vi "COMN-RS232_XBEE_RPI.vi"() -> ()   [LabVIEW 2020]
uses:
  <vilib>/Instr/_visa.llb/VISA Configure Serial Port (Instr).vi
panel:
  out "0_HORA":string
  in  "Enable Termination\nChar (T)":bool=TRUE
  in  "termination char\n(0xA = '\\n' = LF)":u8=10 format="%.0x"
  in  "flow control (0:none)":u16(ring) items=["None", "XON/XOFF", "RTS/CTS", "XON/XOFF & RTS/CTS", "DTR/DSR", "XON/XOFF & DTR/DSR"]
  in  "timeout (10sec)":u32=10000
  in  "stop bits (10: 1 bit)":u16(ring)=10 items=["1.0"=10, "1.5"=15, "2.0"=20]
  in  "parity (0:none)":enum16{"None", "Odd", "Even", "Mark", "Space"}(ring)
  in  "data bits (8)":u16=8 min=5 max=8 step=1
  in  "baud rate (9600)":u32=9600
  in  "VISA resource name":refnum<visa-resource-name>
  in  "stop":bool
  out "codigo":bool
  out "mensj_recib":bool
  out "error recib":errorcluster
  out "PUERTO_COM":refnum<visa-resource-name>
  in  "Boton_Recibir":bool
  out "Text_Recibir":string
  # "COMUNICACIÓN RS232 RPI-XBEE-PC"
  # "TEXTO A RECIBIR"
  # "(c)2021"
  # "ANDRES R. PHILIPPS BENITEZ"
  # "HABILITAR \nCARACTER DE\nTERMINACIÓN"
  # "CARACTER DE\nTERMINACION"
  # "TIMEOUT"
  # "CONTROL DE FLUJO"
  # "BITS DATOS"
  # "PARIDAD"
  # "BITS DE STOP"
  # "BAUDIOS"
  # "PUERTO COM"
  # "CÓDIGO"
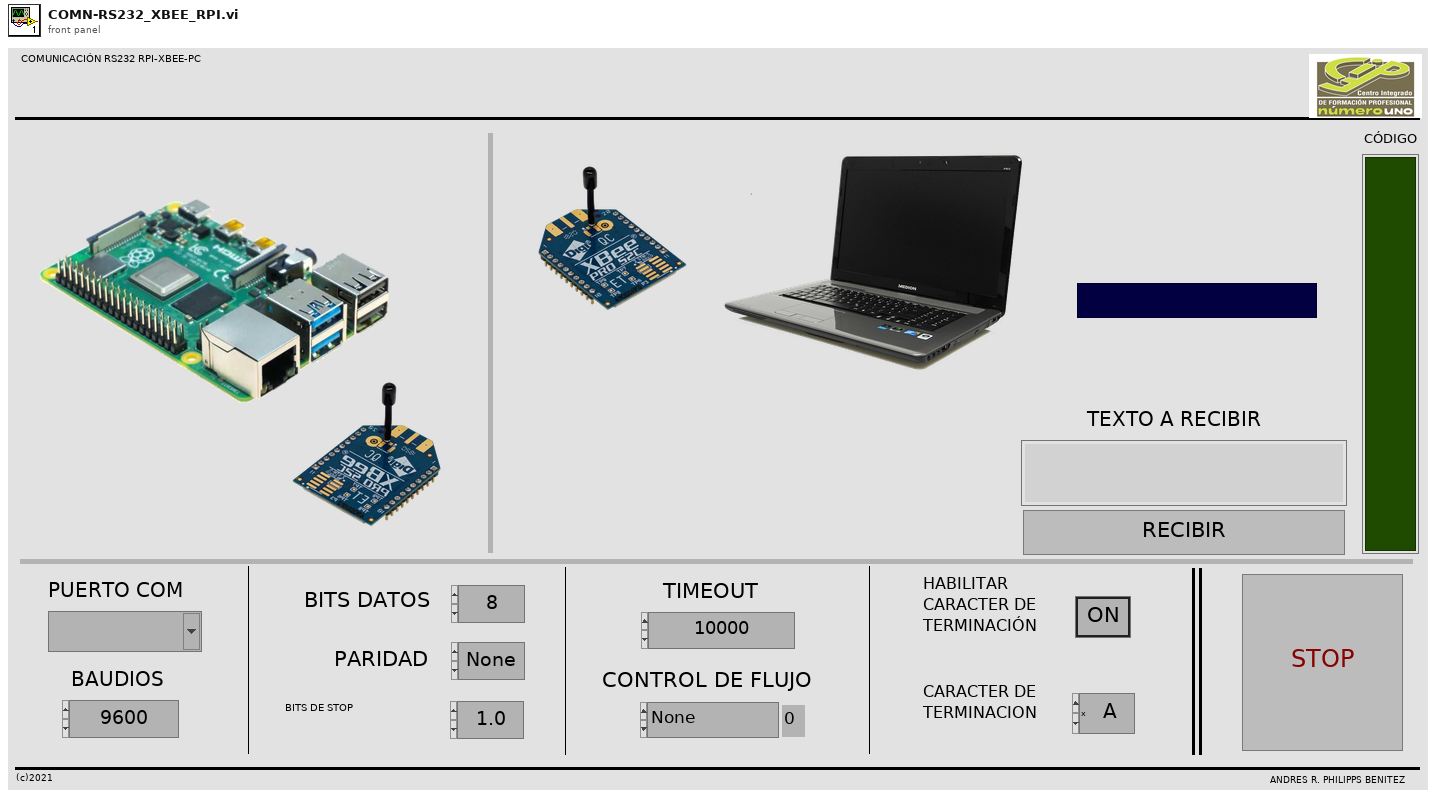
[diagram p1: front panel]
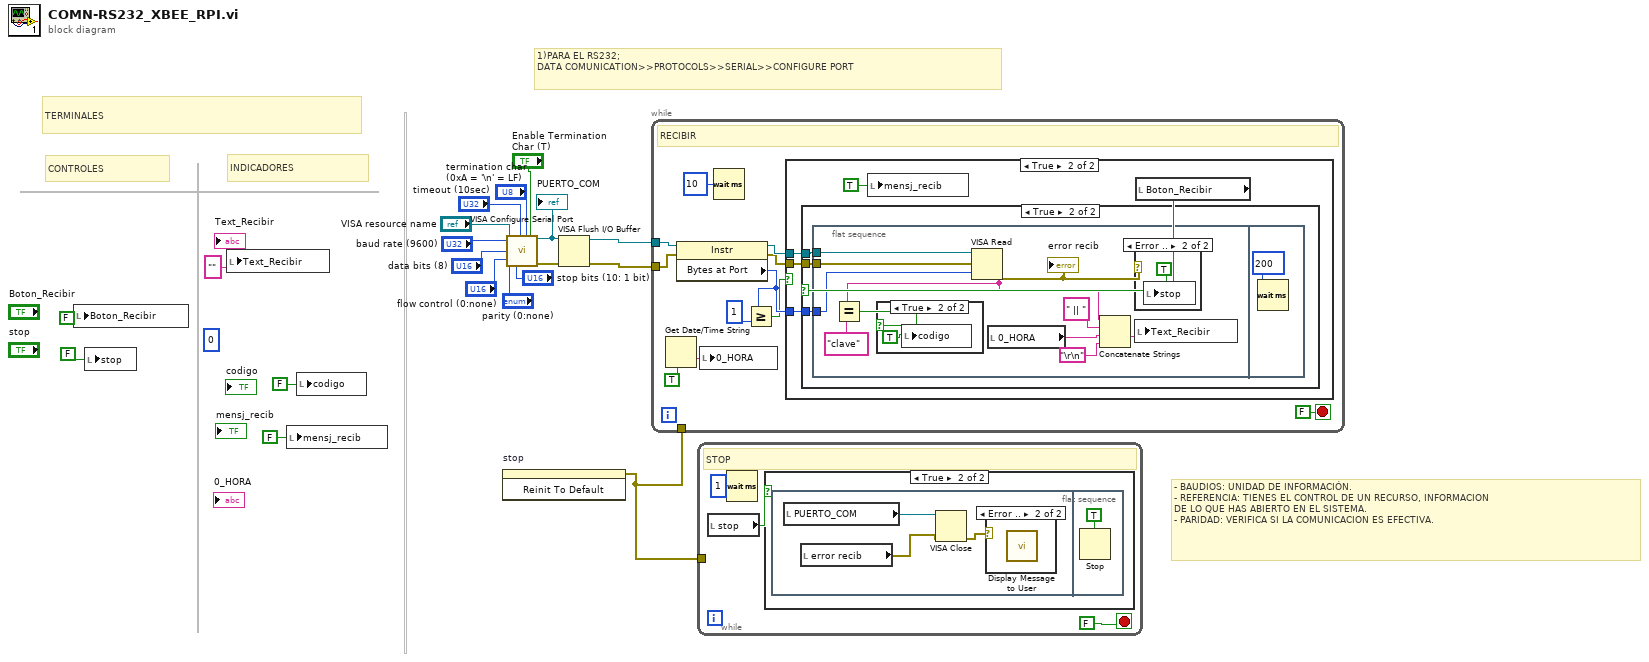
[diagram p0: block diagram]
diagram:
  (unwired) u32 0 ("return count")
  # "- BAUDIOS: UNIDAD DE INFORMACIÓN.\n- REFERENCIA: TIENES EL CONTROL DE UN RECURSO, INFORMACION \nDE LO QUE HAS ABIERTO EN EL SISTEMA.\n- PARIDAD: VERIFICA SI LA COMUNICACION ES EFECTIVA."
  # "1)PARA EL RS232;\nDATA COMUNICATION>>PROTOCOLS>>SERIAL>>CONFIGURE PORT"
  # "INDICADORES"
  # "CONTROLES"
  # "TERMINALES"
  n1 = local write "Boton_Recibir"(FALSE ("Boton_Recibir")) -> ()
  n2 = local write "stop"(FALSE ("stop")) -> ()
  n3 = local write "Text_Recibir"("" ("Text_Recibir")) -> ()
  n4 = local write "mensj_recib"(FALSE ("mensj_recib")) -> ()
  n5 = local write "codigo"(FALSE ("codigo")) -> ()
  n6 = invoke on="stop" class="Bool (strict)" method="Reinit To Default"() -> (error out=w1:errorcluster)  [unwired: 3 in, 2 out]
  n7 = call-poly "VISA Configure Serial Port"("VISA resource name"="VISA resource name", "timeout (10sec)"="timeout (10sec)", "termination char\n(0xA = '\\n' = LF)"="termination char\n(0xA = '\\n' = LF)", "Enable Termination\nChar (T)"="Enable Termination\nChar (T)", "baud rate (9600)"="baud rate (9600)", "data bits (8)"="data bits (8)", "parity (0:none)"="parity (0:none)", "stop bits (10: 1 bit)"="stop bits (10: 1 bit)", "flow control (0:none)"="flow control (0:none)") -> ("VISA resource name out"=w5:refnum<visa-resource-name>, "error out"=w4:errorcluster)  [unwired: 5 in]
  "PUERTO_COM" <- w5
  n8 = VISA Flush I/O Buffer(VISA resource name=w5, error in (no error)=w4) -> (VISA resource name out=w3:refnum<visa-resource-name>, error out=w2:errorcluster)  [unwired: 1 in]
  n9 = while {
    tunnel: w3 -> [w23]
    tunnel: w2 -> [w22]
    tunnel: w1 -> [_]
    stop <- FALSE stop-if-true
    # "RECIBIR"
    n10 = Get Date/Time String(want seconds? (F)=TRUE) -> (time string=w21:string)  [unwired: 2 in, 1 out]
    n11 = property class="Instr"(reference=w23, error in=w22) -> (reference out=w28:refnum<visa-resource-name>, error out=w27:errorcluster, "Bytes at Port"=w26:u32)
    n12 = local write "0_HORA"(w21) -> ()
    n13 = Wait (ms)(milliseconds to wait=u32 10) -> ()  [unwired: 1 out]
    n14 = Greater Or Equal?(x=w26, y=u32 1) -> (x >= y?=w24:bool)
    n15 = case shown="True" w24 {
      tunnel: w28 -> [_ w33]
      tunnel: w27 -> [_ w32]
      tunnel: w26 -> [_ w31]
      frame False {
      }
      frame True {
        n16 = local write "mensj_recib"(TRUE ("mensj_recib")) -> ()
        n17 = local read "Boton_Recibir"() -> (w35:bool)
        n18 = case shown="True" w35 {
          tunnel: w33 -> [_ w38]
          tunnel: w32 -> [_ w37]
          tunnel: w31 -> [_ w36]
          frame False {
          }
          frame True {
            n19 = flat-sequence {
              tunnel: w38 -> [w45]
              tunnel: w37 -> [w44]
              tunnel: w36 -> [w43]
              frame #0 {
                n20 = VISA Read(VISA resource name=w45, byte count=w43, error in (no error)=w44) -> (read buffer=w40:string, error out=w48:errorcluster)  [unwired: 2 out]
                "error recib" <- w48
                n21 = Equal?(x=w40, y="clave") -> (x = y?=w46:bool)
                n22 = case shown="True" w46 {
                  frame False {
                  }
                  frame True {
                    n23 = local write "codigo"(TRUE ("codigo")) -> ()
                  }
                }
                n24 = local read "0_HORA"() -> (w39:string)
                n25 = Concatenate Strings(w40, " || " ("Text_Recibir"), w39, "\r\n") -> (w49:string)
                n26 = case shown="Error .." w48 {
                  frame No Error {
                  }
                  frame Error {
                    n27 = local write "stop"(TRUE ("stop")) -> ()
                  }
                }
                n28 = local write "Text_Recibir"(w49) -> ()
              }
              frame #1 {
                n29 = Wait (ms)(milliseconds to wait=u32 200) -> ()  [unwired: 1 out]
              }
            }
          }
        }
      }
    }
  }
  n30 = while {
    tunnel: w1 -> [_]
    stop <- FALSE stop-if-true
    # "STOP"
    n31 = local read "stop"() -> (w53:bool)
    n32 = Wait (ms)(milliseconds to wait=u32 1) -> ()  [unwired: 1 out]
    n33 = case shown="True" w53 {
      frame False {
      }
      frame True {
        n34 = flat-sequence {
          frame #0 {
            n35 = local read "PUERTO_COM"() -> (w58:refnum<visa-resource-name>)
            n36 = local read "error recib"() -> (w56:errorcluster)
            n37 = VISA Close(VISA resource name=w58, error in (no error)=w56) -> (error out=w57:errorcluster)
            n38 = case shown="Error .." w57 {
              frame No Error {
              }
              frame Error {
                n39 = call "Display Message to User"() -> ()  [unwired: 10 in, 2 out]
              }
            }
          }
          frame #1 {
            n40 = Stop(stop? (T)=TRUE) -> ()
          }
        }
      }
    }
  }
